vi "Read Configuration Parameter.vi"(8 "error in (no error)":errorcluster, 11 "RandomNumberLogger in":refnum<class "RandomNumberLogger.lvclass">) -> (0 "error out":errorcluster, 2 "Configuration":T1, 3 "RandomNumberLogger out":refnum<class "RandomNumberLogger.lvclass">)   [LabVIEW 2020, in "RandomNumberLogger.lvlib" / "RandomNumberLogger.lvclass"]
doc: "<b>Read Configuration Parameter</b>\nThis method returns the configuration parameter from the class data for this plugin. It is returned as a populated <b>Configuration.ctl</b> from this plugin."
uses:
  RandomNumberLogger.lvclass
  C:/Program Files/National Instruments/LabVIEW 2020/vi.lib/FlexLogger/SDK/PluginSDK.lvlibp/PEFClasses/SDK/Processing Element/Processing Element.lvclass
  Configuration.ctl
  Get Configuration Version.vi
  Mutate Configuration to Current.vi
  Default Configuration Parameters.vi
  <vilib>/FlexLogger/SDK/PluginSDK.lvlibp/PEFClasses/SDK/Processing Element/Read Parameters Property.vi
  <vilib>/FlexLogger/SDK/PluginSDK.lvlibp/PEFClasses/SDK/Parameters/PolyHelpers/GetParameter(String).vi
  <vilib>/ADAS Record/Utilities/Config/Data Converter/Populate Container from JSON.vi
  <vilib>/FlexLogger/SDK/PluginSDK.lvlibp/PEFClasses/SDK/Parameters/Parameters.lvclass
panel:
  # "#via_ignore"
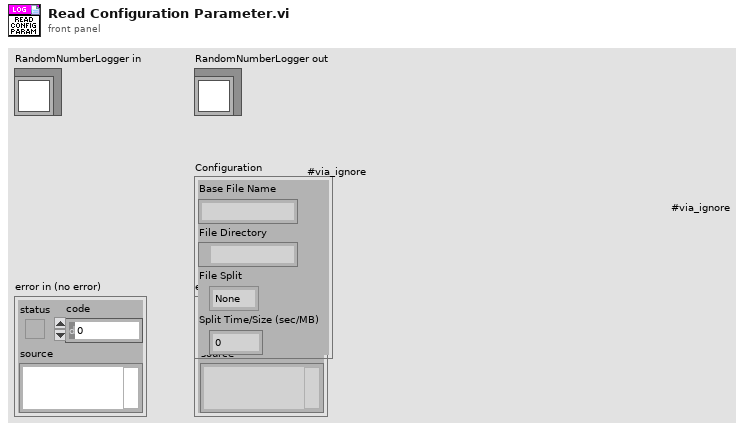
[diagram p1: front panel]
types:
  T1 = typedef "RandomNumberLogger.lvlib/RandomNumberLogger.lvclass/Configuration.ctl" = cluster{"Base File Name":string, "File Directory":path, "File Split":enum16{"None", "Time", "Size"}, "Split Time/Size (sec/MB)":dbl}
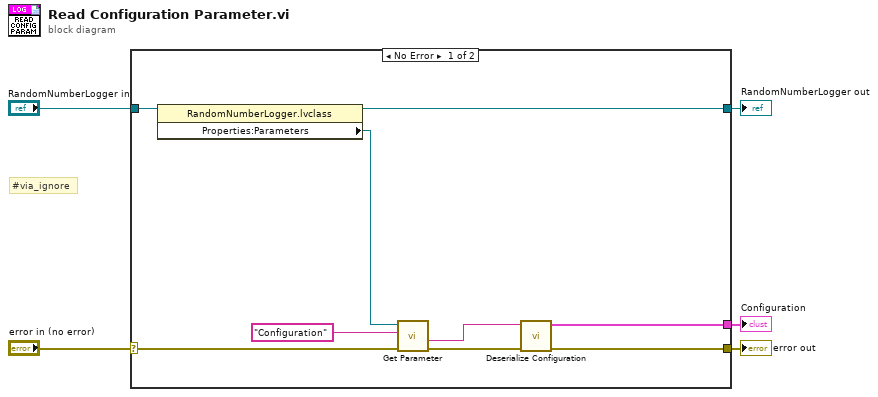
[diagram p0: block diagram]
diagram:
  # "#via_ignore"
  n1 = case shown="No Error" "error in (no error)" {
    selector: "error in (no error)" -> [w8 w16]
    tunnel: [w7 w16] -> w4
    tunnel: [w9 w15] -> w2
    tunnel: "RandomNumberLogger in" -> [w10 w15]
    tunnel: [w6 _] -> w1
    frame No Error {
      n2 = property on="Property Node" class="RandomNumberLogger.lvclass"(reference=w10) -> (reference out=w9:refnum<class "RandomNumberLogger.lvclass">, "Properties:Parameters"=w14:refnum<class "Parameters.lvclass">)  [unwired: 1 in, 1 out]
      n3 = call-poly <vilib>:"Get Parameter.vi"("error in (no error)"=w8, "Name"="Configuration", "Parameters in"=w14) -> ("error out"=w12:errorcluster, "Value"=w11:string)  [unwired: 5 in, 2 out]
      n4 = call "Deserialize Configuration.vi"("error in (no error)"=w12, "Serialized Configuration"=w11) -> ("error out"=w7:errorcluster, "Configuration"=w6:T1)  [unwired: 8 in]
    }
    frame Error {
    }
  }
  "error out" <- w4
  "RandomNumberLogger out" <- w2
  "Configuration" <- w1
